vi "Reset Device Core.vi"(8 "error in (no error)":errorcluster, 11 "IVI_DCPwr in":refnum<class "IVI_DCPwr.lvclass">) -> (0 "error out":errorcluster, 3 "IVI_DCPwr out":refnum<class "IVI_DCPwr.lvclass">)   [LabVIEW 2015, in "IVI_DCPwr.lvlib" / "IVI_DCPwr.lvclass"]
doc: "Perform reset of device."
uses:
  IVI_DCPwr.lvclass
  IVI_DCPwr.lvclass/IVI_DCPwr.ctl
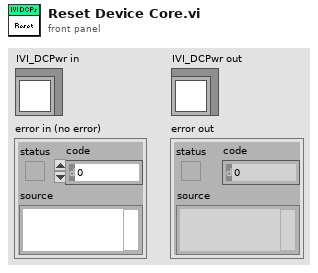
[diagram p1: front panel]
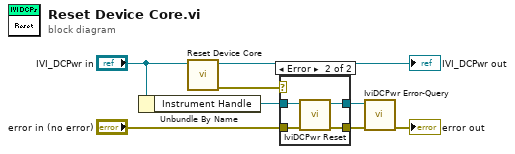
[diagram p0: block diagram]
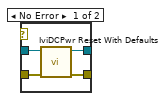
[diagram p2: hidden frame]
diagram:
  n1 = Unbundle By Name("IVI_DCPwr in") -> ("Instrument Handle"=w8:refnum<k15>)
  n2 = call-dynamic "Reset Device Core.vi"("IVI_DCPwr in"="IVI_DCPwr in") -> ("error out"=w1:errorcluster, "IVI_DCPwr out"=→"IVI_DCPwr out":refnum<class "IVI_DCPwr.lvclass">)  [unwired: 9 in]
  n3 = case shown="Error" w1 {
    tunnel: w8 -> [w12 w15]
    tunnel: "error in (no error)" -> [w11 w16]
    tunnel: [w10 w14] -> w6
    tunnel: [w9 w13] -> w5
    frame No Error {
      n4 = call <vilib>:"IviDCPwr Reset With Defaults.vi"("error in (no error)"=w11, "instrument handle"=w12) -> ("error out"=w10:errorcluster, "instrument handle out"=w9:refnum<k15>)  [unwired: 8 in]
    }
    frame Error {
      n5 = call <vilib>:"IviDCPwr Reset.vi"("error in (no error)"=w16, "instrument handle"=w15) -> ("error out"=w14:errorcluster, "instrument handle out"=w13:refnum<k15>)  [unwired: 8 in]
    }
  }
  n6 = call <vilib>:"IviDCPwr Error-Query.vi"("error in (no error)"=w6, "instrument handle"=w5) -> ("error out"=→"error out":errorcluster)  [unwired: 6 in, 3 out]
